vi "practice 3.vi"() -> ()   [LabVIEW 2018]
panel:
  out "クラスタ 2":cluster{"数値":dbl, "ブール":bool, "メーター":dbl} {"メーター" scale=0.0..10.0}
  in  "クラスタ":cluster{"数値":dbl, "ブール":bool, "メーター":dbl} {"メーター" scale=0.0..10.0}
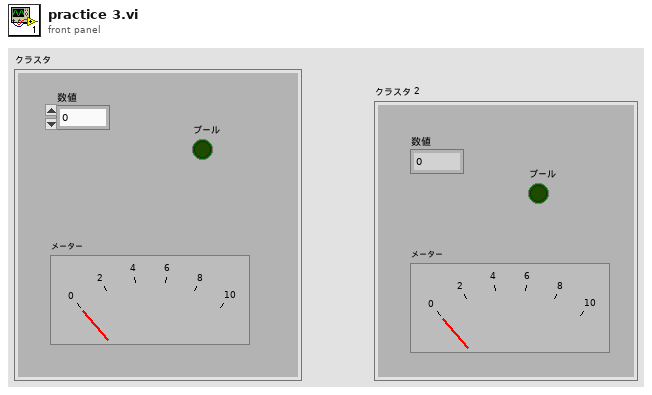
[diagram p1: front panel]
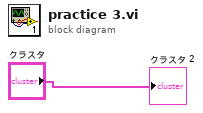
[diagram p0: block diagram]
diagram:
  "クラスタ 2" <- "クラスタ"
